vi "32xx_Config_USB.vi"(7 "Taille buffer d'entrée":u32=64, 8 "entrée d'erreur":errorcluster caption="entrée d'erreur (pas d'erreur)", 10 "TimeOut (ms)":u32=6500, 11 "Port Entrée":refnum<visa-resource-name>="COM1") -> (0 "sortie d'erreur":errorcluster, 3 "Port Sortie":refnum<visa-resource-name>="COM1")   [LabVIEW 2020]
doc: "Configuration du port COM en USB : TimeOut, Taille buffers, etc.."
panel:
  # "© 2008 2020 elc  ALL RIGHTS RESERVED."
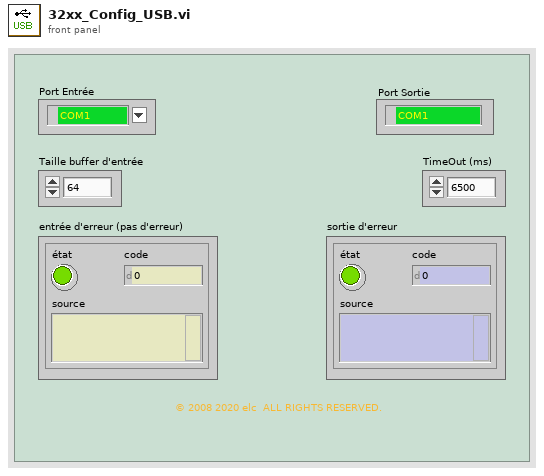
[diagram p1: front panel]
types:
  T1 = typedef "32xx_VISA_Set_IO_Buffer_Mask_Custom.ctl" = u16
  T2 = typedef "32xx_VISA_Flush_IO_BuffMask_Custom.ctl" = u16
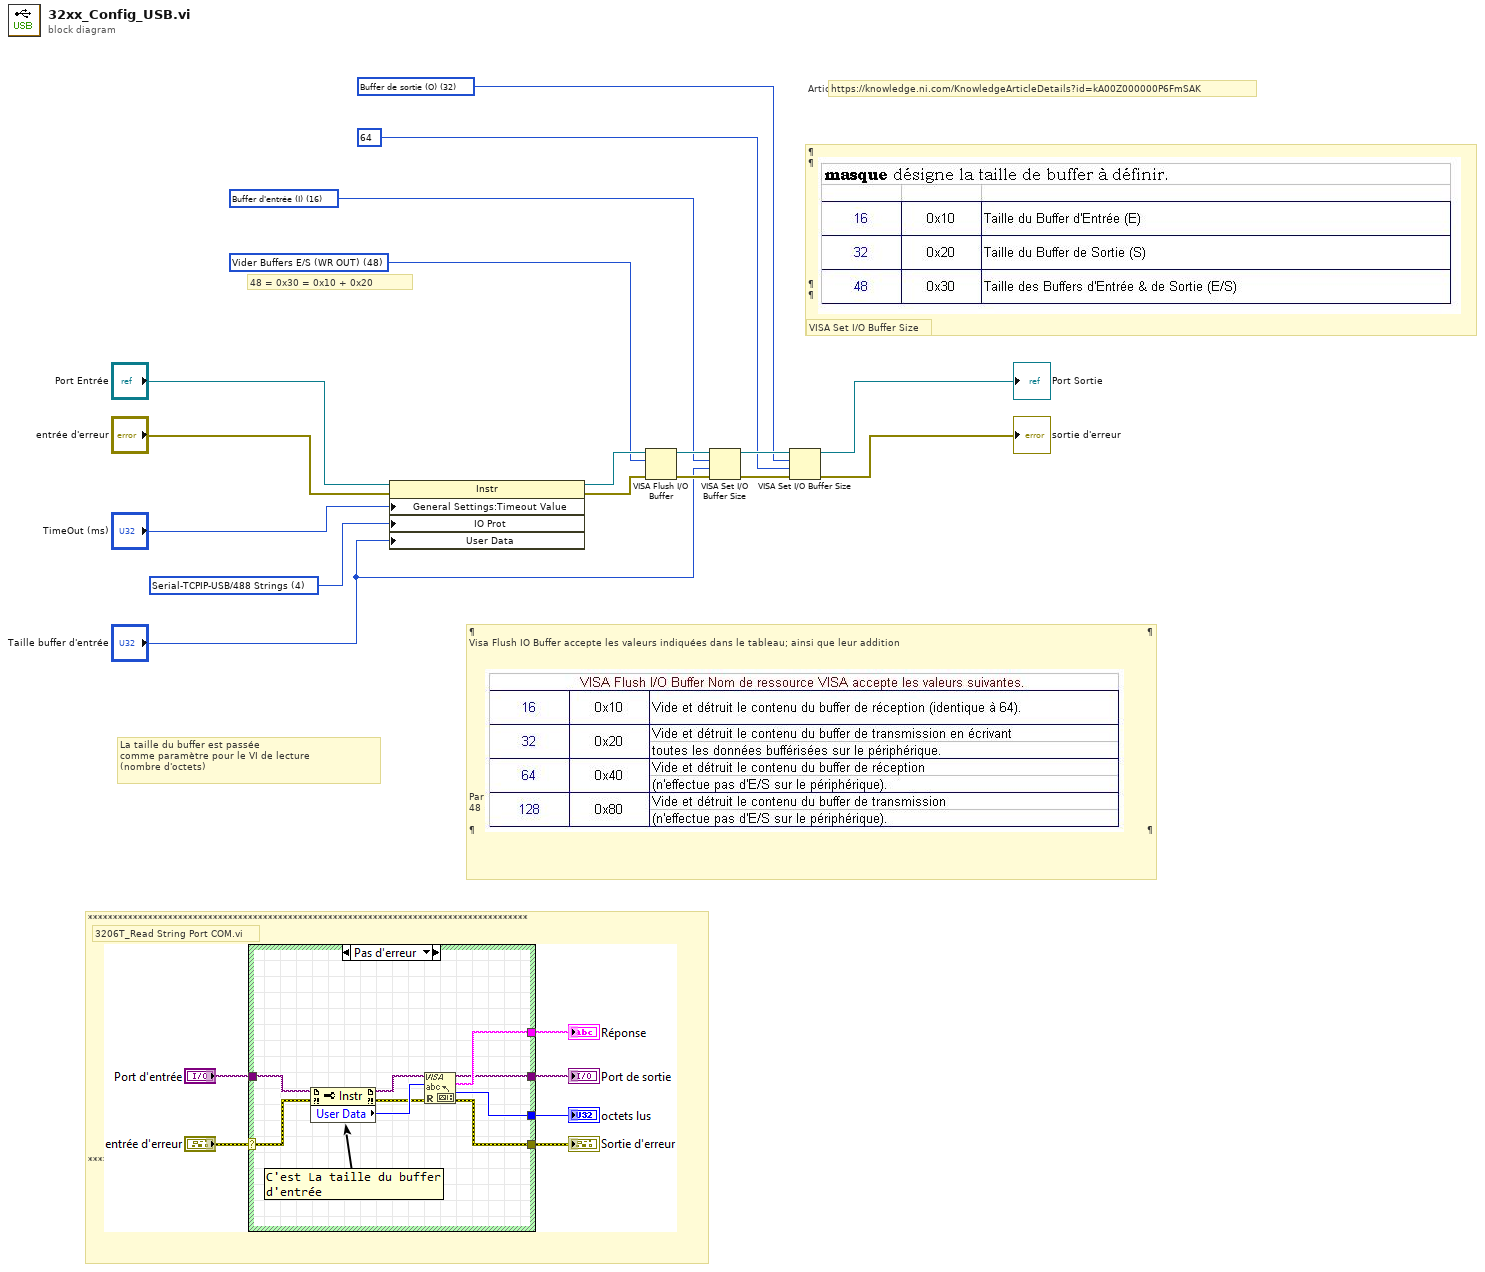
[diagram p0: block diagram]
diagram:
  w1 = T1 32 items=["Buffer d'entrée (I)"=16, "Buffer de sortie (O)"=32, "Buffer d'entrée et de sorties (I/O)"=48] ("Mask")
  w3 = T2 48 items=["Vider le buffer d'entrée"=16, "Écrire le buffer de sortie sur le périphérique"=32, "Vider Buffers E/S (WR OUT)"=48, "Vider le buffer d'entrée (Pas d'E/S)"=64, "Vider le buffer de sortie  (sans écrire)"=128, "Vider les buffers E/S  (Pas d'E/S)"=192] ("Mask")
  w5 = u16 4 items=["Normal"=1, "VXI/FDC"=2, "GPIB/HS488"=3, "Serial-TCPIP-USB/488 Strings"=4, "USBTMC/Vendor-Specific"=5] ("Message Based Settings:IO Protocol")
  w2 = T1 16 items=["Buffer d'entrée (I)"=16, "Buffer de sortie (O)"=32, "Buffer d'entrée et de sorties (I/O)"=48] ("Mask")
  # "3206T_Read String Port COM.vi"
  # "****************************************************************************************\n\n\n\n\n\n\n\n\n\n\n\n\n\n\n\n\n\n\n\n\n\n****************************************************************************************"
  # "La taille du buffer est passée\ncomme paramètre pour le VI de lecture\n(nombre d'octets)"
  # "48 = 0x30 = 0x10 + 0x20"
  # "https://knowledge.ni.com/KnowledgeArticleDetails?id=kA00Z000000P6FmSAK"
  # "Article de labView au sujet  de l'erreur  -1073807298 & du Flush automatique :"
  # "VISA Set I/O Buffer Size"
  # "¶                                                                                                                                                                                                                               ¶\n\n\n\n\n\n\n\n\n\n\n¶                                                                                                                                                                                                                               ¶"
  # "¶                                                                                                                                                                                                                                ¶\nVisa Flush IO Buffer accepte les valeurs indiquées dans le tableau; ainsi que leur addition\n\n\n\n\n\n\n\n\n\n\n\n\n\nPar exemple, la valeur 192 = 128+64 (0xC0 = 0x40 + 0x80)  videra les buffers d'entrée & de sortie, sans écrire sur le périphérique.\n48 = 0x30 = 0x10 + 0x20\n\n¶                                                                                                                                                                                                                                ¶"
  n1 = property class="Instr"(reference="Port Entrée", error in="entrée d'erreur", "General Settings:Timeout Value"="TimeOut (ms)", "IO Prot"=w5, "User Data"="Taille buffer d'entrée") -> (reference out=w14:refnum<visa-resource-name>, error out=w12:errorcluster)
  n2 = VISA Flush I/O Buffer(VISA resource name=w14, mask (16)=w3, error in (no error)=w12) -> (VISA resource name out=w13:refnum<visa-resource-name>, error out=w11:errorcluster)
  n3 = VISA Set I/O Buffer Size(VISA resource name=w13, mask (16)=w2, size (4096)="Taille buffer d'entrée", error in (no error)=w11) -> (VISA resource name out=w10:refnum<visa-resource-name>, error out=w9:errorcluster)
  n4 = VISA Set I/O Buffer Size(VISA resource name=w10, mask (16)=w1, size (4096)=u32 64 ("taille (4096)"), error in (no error)=w9) -> (VISA resource name out=→"Port Sortie":refnum<visa-resource-name>, error out=→"sortie d'erreur":errorcluster)
